vi "水样测试.vi"(10 "数据标记表":string(combo)="N", 11 "水样测试时间":dbl=1.0) -> ()   [LabVIEW 2016, in "斯坦道多参数.lvlib"]
panel:
  out "运行状态":u16(ring) items=["空闲", "水样测试", "标样核查"]
  out "多参数运行日志":string
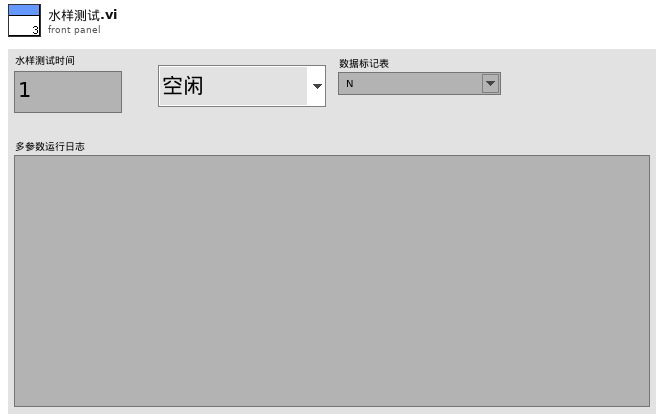
[diagram p1: front panel]
types:
  T1 = cluster{"因子编码":string, "单位":string, "标样参考值":sgl, "水样数据时间":timestamp, "水样实测值":sgl, "水样数据标识":string, "探头温度":sgl}
  T2 = cluster{"温度测量值":sgl, "DO%":sgl, "DOmg/L":sgl, "温度偏移修正值":sgl}
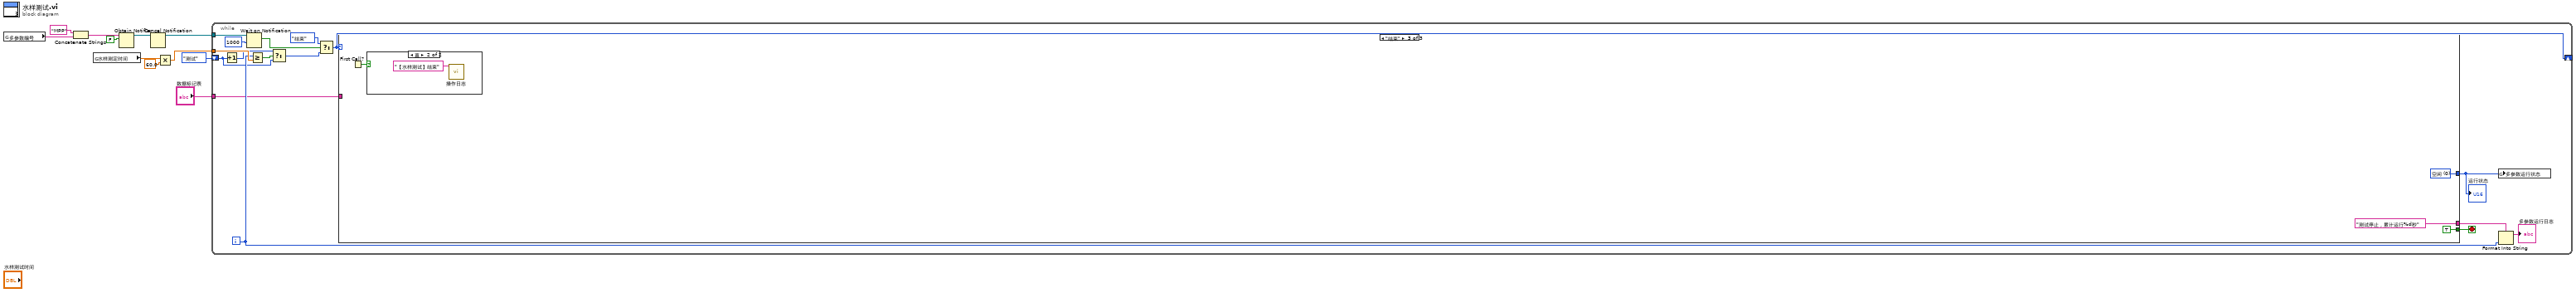
[diagram p0: block diagram]
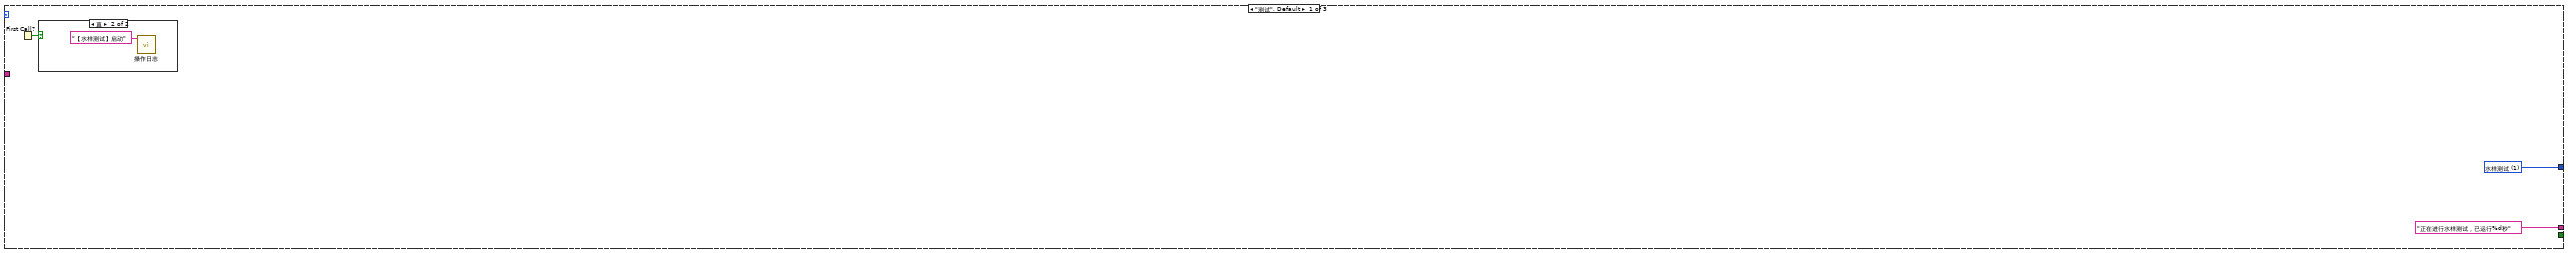
[diagram p2: hidden frame]
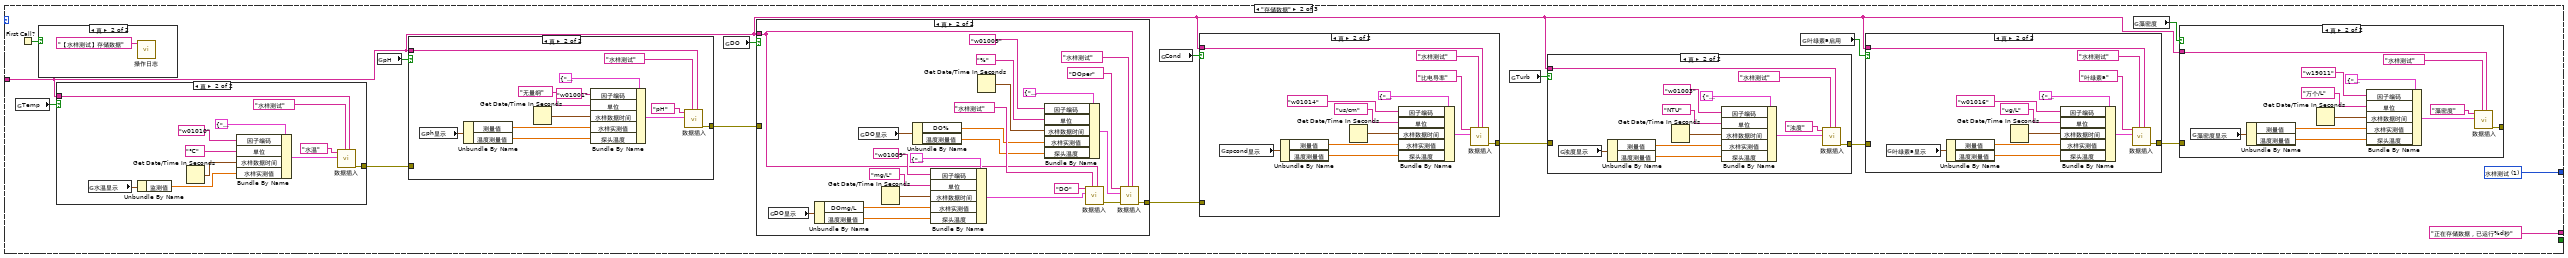
[diagram p4: hidden frame]
diagram:
  n1 = global read "多参数全局变量.vi" "多参数编号"() -> (w2:string)
  n2 = Concatenate Strings("MPP" ("名称（未命名）"), w2) -> (w3:string)
  n3 = global read "断电保存变量.vi" "水样测定时间"() -> (w1:dbl)
  n4 = Obtain Notifier(name (unnamed)=w3, notification data type=FALSE) -> (notifier out=w6:refnum<notifier>)  [unwired: 2 in, 2 out]
  n5 = Cancel Notification(0:w6) -> (8:w5:refnum<notifier>)  [unwired: 1 in, 2 out]
  n6 = Multiply(x=w1, y=60.0) -> (x*y=w10:dbl)
  n7 = while {
    tunnel: w10 -> [w27]
    shift-right: [w14] -> _
    shift-left: enum16{"测试", "存储数据", "结束"}."测试" ("枚举") -> [w21]
    tunnel: w5 -> [w19]
    tunnel: "数据标记表" -> [w13]
    i -> [w25]
    stop <- w26 stop-if-true
    n8 = Increment(x=w21) -> (x+1=w20:enum16{"测试", "存储数据", "结束"})
    n9 = Wait on Notification(notifier=w19, timeout in ms (-1)=1000 ("超时毫秒(-1)")) -> (notification=w17:bool)  [unwired: 2 in, 3 out]
    n10 = Greater Or Equal?(x=w25, y=w27) -> (x >= y?=w22:bool)
    n11 = Select(t=w20, s=w22, f=w21) -> (s? t:f=w15:enum16{"测试", "存储数据", "结束"})
    n12 = Select(t=enum16{"测试", "存储数据", "结束"}."结束" ("枚举"), s=w17, f=w15) -> (s? t:f=w14:enum16{"测试", "存储数据", "结束"})
    n13 = case shown="\"结束\"" w14 {
      tunnel: [_ _ TRUE] -> w26
      tunnel: ["正在进行水样测试，已运行%d秒" ("格式字符串") "正在存储数据，已运行%d秒" ("格式字符串") "测试停止，累计运行%d秒" ("格式字符串")] -> w24
      tunnel: [w29 w36 w145] -> w12
      tunnel: w13 -> [_ w35 _]
      frame "测试", Default {
        w29 = u16 1 items=["空闲", "水样测试", "标样核查"] ("多参数运行状态")
        n14 = First Call?() -> (First Call?: T/F=w28:bool)
        n15 = case shown="真" w28 {
          frame False {
          }
          frame True {
            n16 = call "操作日志.vi"("日志信息"="【水样测试】启动") -> ()  [unwired: 10 in, 1 out]
          }
        }
      }
      frame "存储数据" {
        w36 = u16 1 items=["空闲", "水样测试", "标样核查"] ("多参数运行状态")
        n17 = global read "断电保存变量.vi" "Temp"() -> (w43:bool)
        n18 = First Call?() -> (First Call?: T/F=w32:bool)
        n19 = case shown="真" w32 {
          frame False {
          }
          frame True {
            n20 = call "操作日志.vi"("日志信息"="【水样测试】存储数据") -> ()  [unwired: 10 in, 1 out]
          }
        }
        n21 = case shown="真" w43 {
          tunnel: [_ w136] -> w38
          tunnel: w35 -> [_ w135]
          frame False {
          }
          frame True {
            n22 = global read "多参数全局变量.vi" "水温显示"() -> (w134:cluster{"CH":u16, "监测值":dbl, "温度偏移修正值":sgl})
            n23 = Unbundle By Name(w134) -> ("监测值"=w133:dbl)
            n24 = Get Date/Time In Seconds() -> (seconds since 1Jan1904=w142:timestamp)
            n25 = Bundle By Name(cluster=T1 {"因子编码"="w01003", "单位"="无量纲", "标样参考值"=0.0, "水样数据时间"=timestamp(0 s since 1904-01-01), "水样实测值"=0.0, "水样数据标识"="N", "探头温度"=0.0} ("data in"), "因子编码"="w01010", "单位"="℃", "水样数据时间"=w142, "水样实测值"=w133) -> (w141:T1)
            n26 = call "数据插入.vi"("数据标记表"=w135, "测量模式"="水样测试", "data in"=w141, "table输入"="水温") -> ("error out"=w136:errorcluster)  [unwired: 7 in]
          }
        }
        n27 = global read "断电保存变量.vi" "pH"() -> (w44:bool)
        n28 = case shown="真" w44 {
          tunnel: w38 -> [_ _]
          tunnel: [_ w125] -> w39
          tunnel: w35 -> [_ w124]
          frame False {
          }
          frame True {
            n29 = global read "多参数全局变量.vi" "ph显示"() -> (w123:cluster{"温度测量值":sgl, "测量值":sgl, "温度偏移修正值":sgl})
            n30 = Unbundle By Name(w123) -> ("测量值"=w122:sgl, "温度测量值"=w121:sgl)
            n31 = Get Date/Time In Seconds() -> (seconds since 1Jan1904=w130:timestamp)
            n32 = Bundle By Name(cluster=T1 {"因子编码"="w01003", "单位"="无量纲", "标样参考值"=0.0, "水样数据时间"=timestamp(0 s since 1904-01-01), "水样实测值"=0.0, "水样数据标识"="N", "探头温度"=0.0} ("data in"), "因子编码"="w01001", "单位"="无量纲", "水样数据时间"=w130, "水样实测值"=w122, "探头温度"=w121) -> (w131:T1)
            n33 = call "数据插入.vi"("数据标记表"=w124, "测量模式"="水样测试", "data in"=w131, "table输入"="pH") -> ("error out"=w125:errorcluster)  [unwired: 7 in]
          }
        }
        n34 = global read "断电保存变量.vi" "DO"() -> (w45:bool)
        n35 = case shown="真" w45 {
          tunnel: w39 -> [_ _]
          tunnel: [_ w113] -> w40
          tunnel: w35 -> [_ w111]
          frame False {
          }
          frame True {
            n36 = global read "多参数全局变量.vi" "DO显示"() -> (w102:T2)
            n37 = Unbundle By Name(w102) -> ("DOmg/L"=w101:sgl, "温度测量值"=w100:sgl)
            n38 = global read "多参数全局变量.vi" "DO显示"() -> (w99:T2)
            n39 = Get Date/Time In Seconds() -> (seconds since 1Jan1904=w119:timestamp)
            n40 = Unbundle By Name(w99) -> ("DO%"=w106:sgl, "温度测量值"=w104:sgl)
            n41 = Bundle By Name(cluster=T1 {"因子编码"="w01003", "单位"="无量纲", "标样参考值"=0.0, "水样数据时间"=timestamp(0 s since 1904-01-01), "水样实测值"=0.0, "水样数据标识"="N", "探头温度"=0.0} ("data in"), "因子编码"="w01009", "单位"="mg/L", "水样数据时间"=w119, "水样实测值"=w101, "探头温度"=w100) -> (w118:T1)
            n42 = Get Date/Time In Seconds() -> (seconds since 1Jan1904=w107:timestamp)
            n43 = Bundle By Name(cluster=T1 {"因子编码"="w01003", "单位"="无量纲", "标样参考值"=0.0, "水样数据时间"=timestamp(0 s since 1904-01-01), "水样实测值"=0.0, "水样数据标识"="N", "探头温度"=0.0} ("data in"), "因子编码"="w01009", "单位"="%", "水样数据时间"=w107, "水样实测值"=w106, "探头温度"=w104) -> (w103:T1)
            n44 = call "数据插入.vi"("数据标记表"=w111, "测量模式"="水样测试", "data in"=w118, "table输入"="DO") -> ("error out"=w98:errorcluster)  [unwired: 7 in]
            n45 = call "数据插入.vi"("数据标记表"=w111, "测量模式"="水样测试", "error in (no error)"=w98, "data in"=w103, "table输入"="DOper") -> ("error out"=w113:errorcluster)  [unwired: 6 in]
          }
        }
        n46 = global read "断电保存变量.vi" "Cond"() -> (w46:bool)
        n47 = case shown="真" w46 {
          tunnel: w40 -> [_ _]
          tunnel: [_ w90] -> w41
          tunnel: w35 -> [_ w89]
          frame False {
          }
          frame True {
            n48 = global read "多参数全局变量.vi" "spcond显示"() -> (w88:cluster{"温度测量值":sgl, "测量值":sgl, "温度偏移修正值":sgl})
            n49 = Unbundle By Name(w88) -> ("测量值"=w87:sgl, "温度测量值"=w86:sgl)
            n50 = Get Date/Time In Seconds() -> (seconds since 1Jan1904=w95:timestamp)
            n51 = Bundle By Name(cluster=T1 {"因子编码"="w01003", "单位"="无量纲", "标样参考值"=0.0, "水样数据时间"=timestamp(0 s since 1904-01-01), "水样实测值"=0.0, "水样数据标识"="N", "探头温度"=0.0} ("data in"), "因子编码"="w01014", "单位"="us/cm", "水样数据时间"=w95, "水样实测值"=w87, "探头温度"=w86) -> (w96:T1)
            n52 = call "数据插入.vi"("数据标记表"=w89, "测量模式"="水样测试", "data in"=w96, "table输入"="比电导率") -> ("error out"=w90:errorcluster)  [unwired: 7 in]
          }
        }
        n53 = global read "断电保存变量.vi" "Turb"() -> (w47:bool)
        n54 = case shown="真" w47 {
          tunnel: w41 -> [_ _]
          tunnel: [_ w78] -> w42
          tunnel: w35 -> [_ w77]
          frame False {
          }
          frame True {
            n55 = global read "多参数全局变量.vi" "浊度显示"() -> (w76:cluster{"温度测量值":sgl, "测量值":sgl, "温度偏移修正值":sgl})
            n56 = Unbundle By Name(w76) -> ("测量值"=w75:sgl, "温度测量值"=w74:sgl)
            n57 = Get Date/Time In Seconds() -> (seconds since 1Jan1904=w84:timestamp)
            n58 = Bundle By Name(cluster=T1 {"因子编码"="w01003", "单位"="无量纲", "标样参考值"=0.0, "水样数据时间"=timestamp(0 s since 1904-01-01), "水样实测值"=0.0, "水样数据标识"="N", "探头温度"=0.0} ("data in"), "因子编码"="w01003", "单位"="NTU", "水样数据时间"=w84, "水样实测值"=w75, "探头温度"=w74) -> (w83:T1)
            n59 = call "数据插入.vi"("数据标记表"=w77, "测量模式"="水样测试", "data in"=w83, "table输入"="浊度") -> ("error out"=w78:errorcluster)  [unwired: 7 in]
          }
        }
        n60 = global read "断电保存变量.vi" "叶绿素a启用"() -> (w48:bool)
        n61 = case shown="真" w48 {
          tunnel: w42 -> [_ _]
          tunnel: [_ w64] -> w33
          tunnel: w35 -> [_ w63]
          frame False {
          }
          frame True {
            n62 = global read "多参数全局变量.vi" "叶绿素a显示"() -> (w62:cluster{"温度测量值":sgl, "测量值":sgl, "温度偏移修正值":sgl})
            n63 = Unbundle By Name(w62) -> ("测量值"=w71:sgl, "温度测量值"=w69:sgl)
            n64 = Get Date/Time In Seconds() -> (seconds since 1Jan1904=w72:timestamp)
            n65 = Bundle By Name(cluster=T1 {"因子编码"="w01003", "单位"="无量纲", "标样参考值"=0.0, "水样数据时间"=timestamp(0 s since 1904-01-01), "水样实测值"=0.0, "水样数据标识"="N", "探头温度"=0.0} ("data in"), "因子编码"="w01016", "单位"="ug/L", "水样数据时间"=w72, "水样实测值"=w71, "探头温度"=w69) -> (w67:T1)
            n66 = call "数据插入.vi"("数据标记表"=w63, "测量模式"="水样测试", "data in"=w67, "table输入"="叶绿素a") -> ("error out"=w64:errorcluster)  [unwired: 7 in]
          }
        }
        n67 = global read "断电保存变量.vi" "藻密度"() -> (w34:bool)
        n68 = case shown="真" w34 {
          tunnel: [_ w52] -> _
          tunnel: w35 -> [_ w51]
          tunnel: w33 -> [_ _]
          frame False {
          }
          frame True {
            n69 = global read "多参数全局变量.vi" "藻密度显示"() -> (w50:cluster{"温度测量值":sgl, "测量值":sgl, "温度偏移修正值":sgl})
            n70 = Unbundle By Name(w50) -> ("测量值"=w59:sgl, "温度测量值"=w57:sgl)
            n71 = Get Date/Time In Seconds() -> (seconds since 1Jan1904=w60:timestamp)
            n72 = Bundle By Name(cluster=T1 {"因子编码"="w01003", "单位"="无量纲", "标样参考值"=0.0, "水样数据时间"=timestamp(0 s since 1904-01-01), "水样实测值"=0.0, "水样数据标识"="N", "探头温度"=0.0} ("data in"), "因子编码"="w19011", "单位"="万个/L", "水样数据时间"=w60, "水样实测值"=w59, "探头温度"=w57) -> (w55:T1)
            n73 = call "数据插入.vi"("数据标记表"=w51, "测量模式"="水样测试", "data in"=w55, "table输入"="藻密度") -> ("error out"=w52:errorcluster)  [unwired: 7 in]
          }
        }
      }
      frame "结束" {
        w145 = u16 0 items=["空闲", "水样测试", "标样核查"] ("多参数运行状态")
        n74 = First Call?() -> (First Call?: T/F=w144:bool)
        n75 = case shown="真" w144 {
          frame False {
          }
          frame True {
            n76 = call "操作日志.vi"("日志信息"="【水样测试】结束") -> ()  [unwired: 10 in, 1 out]
          }
        }
      }
    }
    "运行状态" <- w12
    n77 = global write "多参数全局变量.vi" "多参数运行状态"(w12) -> ()
    n78 = Format Into String(format string=w24, w25) -> (resulting string=→"多参数运行日志":string)  [unwired: 2 in, 1 out]
  }
